vi "Counts to pC_2011.vi"(0 "Z map":dbl[][](array[numeric]), 1 "Screen&Camera 2":T1={"Screen Orientation"="Regular", "Screen angle"="Flat", "Lens"=enum."FL1-f8x08", "Calibration (mm/pix)"=1.0}, 3 "Filter factor":dbl=1.0, 4 "Electron energy (MeV)":dbl=100.0) -> (7 "Counts/pC":dbl[][](array[numeric]))   [LabVIEW 2013]
uses:
  Controls/ScreenCam2_TypDEf_Bella.ctl
  Controls/CamAndObj_TypDEf_Bella.ctl
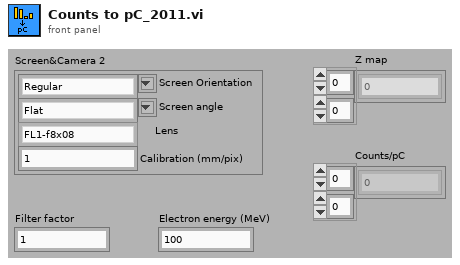
[diagram p1: front panel]
types:
  T1 = typedef "ScreenCam2_TypDEf_Bella.ctl" = cluster{"Screen Orientation":string, "Screen angle":string, "Lens":T2, "Calibration (mm/pix)":dbl}
  T2 = typedef "CamAndObj_TypDEf_Bella.ctl" = enum16{"FL1-f8x08", "FL1-f8x06", "FL1-f8", "ch300-f50", "FL2G-f8", "FL3M14-f8", "FL3M14-f8x08", "FL3M14-f8x08(2x2)"}
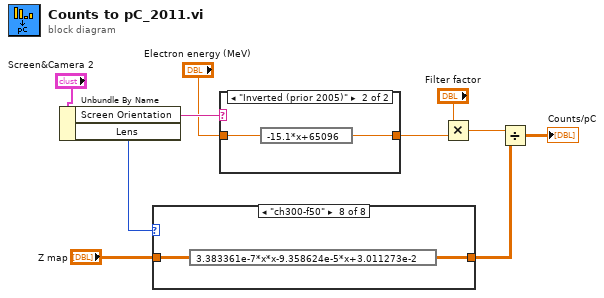
[diagram p0: block diagram]
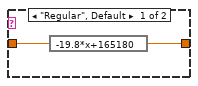
[diagram p2: hidden frame]
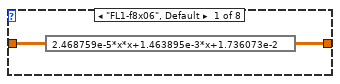
[diagram p3: hidden frame]
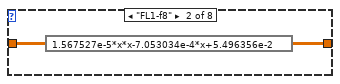
[diagram p4: hidden frame]
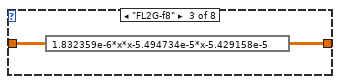
[diagram p5: hidden frame]
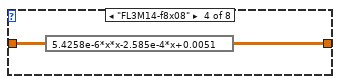
[diagram p6: hidden frame]
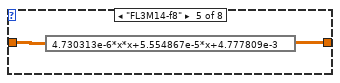
[diagram p7: hidden frame]
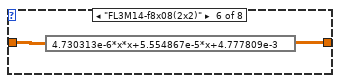
[diagram p8: hidden frame]
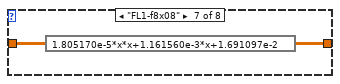
[diagram p9: hidden frame]
diagram:
  n1 = Unbundle By Name("Screen&Camera 2") -> ("Screen Orientation"=w9:string, "Lens"=w7:T2)
  n2 = case shown="\"ch300-f50\"" w7 {
    tunnel: [w12 w14 w16 w18 w20 w22 w24 w26] -> w2
    tunnel: "Z map" -> [w11 w13 w15 w17 w19 w21 w23 w25]
    frame "FL1-f8x06", Default {
      n3 = expression code="2.468759e-5*x*x+1.463895e-3*x+1.736073e-2"(w11) -> (w12:dbl[][])
    }
    frame "FL1-f8" {
      n4 = expression code="1.567527e-5*x*x-7.053034e-4*x+5.496356e-2"(w13) -> (w14:dbl[][])
    }
    frame "FL2G-f8" {
      n5 = expression code="1.832359e-6*x*x-5.494734e-5*x-5.429158e-5"(w15) -> (w16:dbl[][])
    }
    frame "FL3M14-f8x08" {
      n6 = expression code="5.4258e-6*x*x-2.585e-4*x+0.0051"(w17) -> (w18:dbl[][])
    }
    frame "FL3M14-f8" {
      n7 = expression code="4.730313e-6*x*x+5.554867e-5*x+4.777809e-3"(w19) -> (w20:dbl[][])
    }
    frame "FL3M14-f8x08(2x2)" {
      n8 = expression code="4.730313e-6*x*x+5.554867e-5*x+4.777809e-3"(w21) -> (w22:dbl[][])
    }
    frame "FL1-f8x08" {
      n9 = expression code="1.805170e-5*x*x+1.161560e-3*x+1.691097e-2"(w23) -> (w24:dbl[][])
    }
    frame "ch300-f50" {
      n10 = expression code="3.383361e-7*x*x-9.358624e-5*x+3.011273e-2"(w25) -> (w26:dbl[][])
    }
  }
  n11 = case shown="\"Inverted (prior 2005)\"" w9 {
    tunnel: "Electron energy (MeV)" -> [w28 w29]
    tunnel: [w27 w30] -> w5
    frame "Regular", Default {
      n12 = expression code="-19.8*x+165180"(w28) -> (w27:dbl)
    }
    frame "Inverted (prior 2005)" {
      n13 = expression code="-15.1*x+65096"(w29) -> (w30:dbl)
    }
  }
  n14 = Multiply(x="Filter factor", y=w5) -> (x*y=w3:dbl)
  n15 = Divide(x=w3, y=w2) -> (x/y=→"Counts/pC":dbl[][])
